vi "Motor.vi"(1 "Duty Cycle (%) 2":dbl(slide)=50.0 caption="Duty Cycle (%)" min=0.0 max=100.0 step=5.0 scale=0.0..100.0, 2 "Motor Dir 2":bool) -> (0 "DUTY CYCLE":dynamicdata(graph) caption="Square")   [LabVIEW 2010]
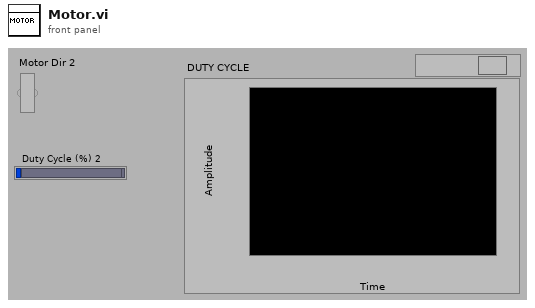
[diagram p1: front panel]
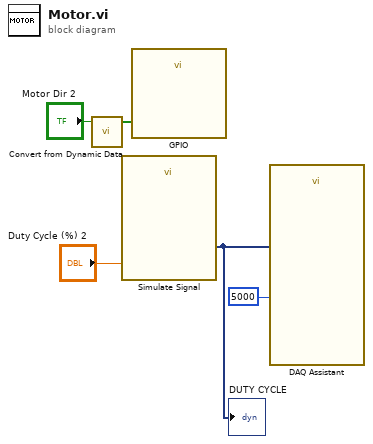
[diagram p0: block diagram]
diagram:
  n1 = call "Convert from Dynamic Data"("Dynamic Data Type"="Motor Dir 2") -> ("Array"=w1:bool[])  [unwired: 3 in]
  n2 = call "Simulate Signal"("Duty Cycle (%)"="Duty Cycle (%) 2") -> ("Square"=w2:dynamicdata)  [unwired: 13 in, 1 out]
  "DUTY CYCLE" <- w2
  n3 = call "GPIO"("data"=w1) -> ()  [unwired: 17 in, 2 out]
  n4 = call "DAQ Assistant"("data"=w2, "rate"=5000) -> ()  [unwired: 15 in, 3 out]
